vi "SetChannelVset.vi"(7 "LabVIEW Web Service Request":refnum<class "Web Request.lvclass">) -> ()   [LabVIEW 2018]
uses:
  <vilib>/wsapi/Web Request.lvclass
  subvis/Channel Properties.ctl
  CAEN globals.vi
panel:
  in  "error in (no error)":errorcluster
  # "Use the Web Service Request input terminal to call the VIs on the Web Services palette. Do not remove it from the connector pane unless you don't need access to the palette."
  # "Each additional control wired to the connector pane will be available as an input in the URL. To include an indicator in terminal-mode output (the default setting), it must also be wired to the connector pane."
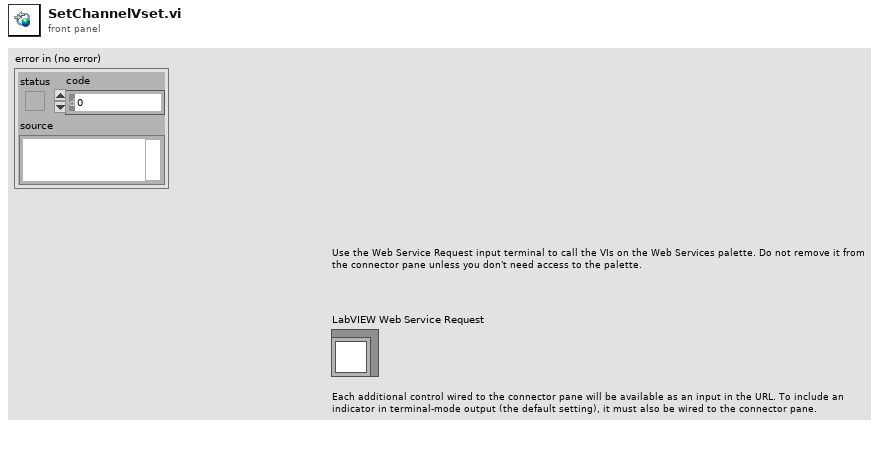
[diagram p1: front panel]
types:
  T1 = typedef "Channel Properties.ctl" = enum16{"Name", "Vset", "Vfile", "Vswmax", "Iset", "Enable", "Flag", "Vbackup"}
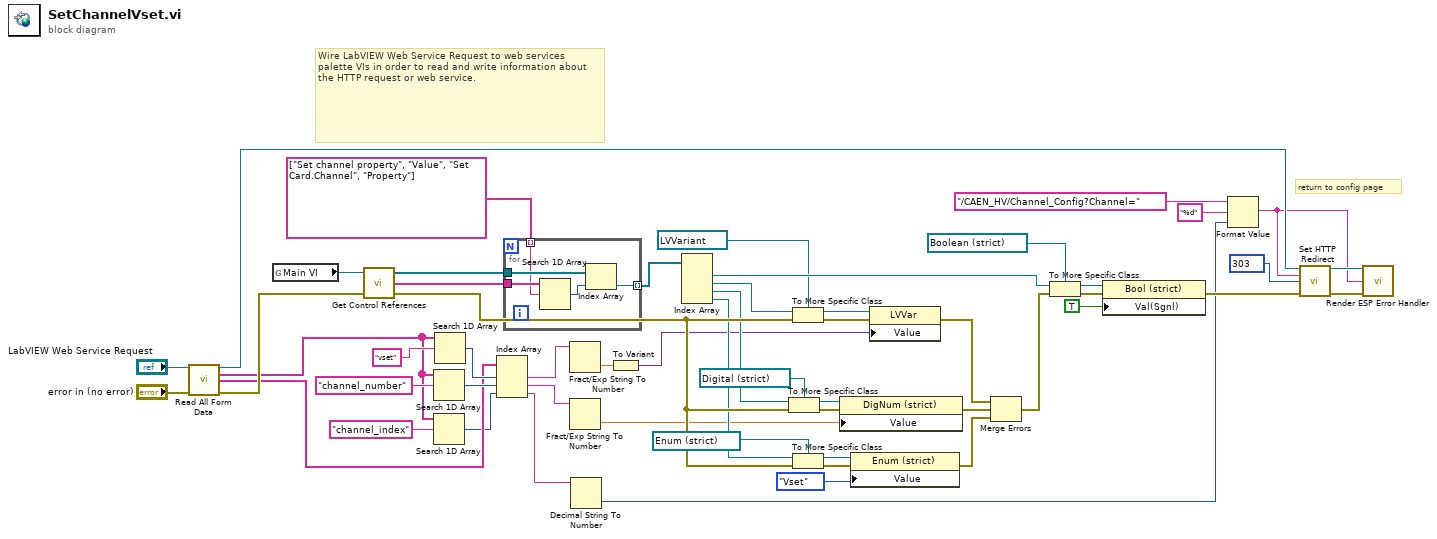
[diagram p0: block diagram]
diagram:
  w49 = 303 items=["100"=100, "101"=101, "200"=200, "201"=201, "202"=202, "203"=203, "204"=204, "205"=205, "206"=206, "300"=300, "301"=301, "302"=302, "303"=303, "304"=304, "305"=305, "306"=306, "307"=307, "400"=400, "401"=401, "402"=402, "403"=403, "404"=404, "405"=405, "406"=406, "407"=407, "408"=408, "409"=409, "410"=410, "411"=411, "412"=412, "413"=413, "414"=414, "415"=415, "416"=416, "417"=417, "500"=500, "501"=501, "502"=502, "503"=503, "504"=504, "505"=505] ("response code (307)")
  # "return to config page"
  # "Wire LabVIEW Web Service Request to web services palette VIs in order to read and write information about the HTTP request or web service."
  n1 = call <vilib>:"Read All Form Data.vi"("LabVIEW Web Service Request"="LabVIEW Web Service Request", "error in (no error)"="error in (no error)") -> ("LabVIEW Web Service Request out"=w25:refnum<class "Web Request.lvclass">, "Key"=w6:string[], "Value"=w17:string[], "error out"=w26:errorcluster)  [unwired: 9 in, 1 out]
  n2 = global read "CAEN globals.vi" "Main VI"() -> (w54:refnum<vi>)
  n3 = call "Get Control References.vi"("error in"=w26, "This vi"=w54) -> ("error out"=w28:errorcluster, "Control Names"=w53:string[], "Controls[]"=w52:refnum<vi>[])  [unwired: 1 in]
  n4 = Search 1D Array(1D array=w6, element="channel_number") -> (index of element=w44:i32)  [unwired: 1 in]
  n5 = Search 1D Array(1D array=w6, element="channel_index") -> (index of element=w5:i32)  [unwired: 1 in]
  n6 = Search 1D Array(1D array=w6, element="vset") -> (index of element=w45:i32)  [unwired: 1 in]
  n7 = Index Array(array=w17, index #1=w45, index #2=w44, index #3=w5) -> (element #1=w16:string, element #2=w13:string, element #3=w4:string)
  n8 = for {
    tunnel: w53 -> [w59]
    tunnel: w52 -> [w58]
    tunnel: [w56] -> w23 mode=indexing
    tunnel: string[] ["Set channel property", "Value", "Set Card.Channel", "Property"] ("Control Names") -> [w55] mode=indexing
    n9 = Search 1D Array(1D array=w59, element=w55) -> (index of element=w57:i32)  [unwired: 1 in]
    n10 = Index Array(array=w58, index=w57) -> (element=w56:refnum<vi>)
  }
  n11 = Fract/Exp String To Number(string=w16) -> (number=w15:dbl)  [unwired: 3 in, 1 out]
  n12 = Fract/Exp String To Number(string=w13) -> (number=w10:dbl)  [unwired: 3 in, 1 out]
  n13 = Decimal String To Number(string=w4) -> (number=w3:i32)  [unwired: 2 in, 1 out]
  n14 = To Variant(anything=w15) -> (Variant=w14:variant)
  n15 = Index Array(array=w23) -> (element #1=w22:refnum<vi>, element #2=w21:refnum<vi>, element #3=w20:refnum<vi>, element #4=w19:refnum<vi>)  [unwired: 4 in]
  n16 = To More Specific Class(target class=refnum<vi> refnum ("number"), reference=w20, error in=w28) -> (specific class reference=w41:refnum<vi>, error out=w40:errorcluster)
  n17 = To More Specific Class(target class=refnum<vi> refnum ("Value"), reference=w21, error in=w28) -> (specific class reference=w50:refnum<vi>, error out=w51:errorcluster)
  n18 = To More Specific Class(target class=refnum<vi> refnum ("Value (Signaling)"), reference=w19, error in=w28) -> (specific class reference=w38:refnum<vi>, error out=w39:errorcluster)
  n19 = property class="DigNum (strict)"(reference=w41, error in=w40, "Value"=w10) -> (error out=w31:errorcluster)  [unwired: 1 out]
  n20 = property class="Enum (strict)"(reference=w38, error in=w39, "Value"=Channel_Properties."Vset" ("Value (Signaling)")) -> (error out=w32:errorcluster)  [unwired: 1 out]
  n21 = property class="LVVar"(reference=w50, error in=w51, "Value"=w14) -> (error out=w30:errorcluster)  [unwired: 1 out]
  n22 = Merge Errors(w30, w31, w32) -> (w29:errorcluster)
  n23 = To More Specific Class(target class=refnum<vi> refnum ("replace all? (F)"), reference=w22, error in=w29) -> (specific class reference=w36:refnum<vi>, error out=w35:errorcluster)
  n24 = property class="Bool (strict)"(reference=w36, error in=w35, "Val(Sgnl)"=TRUE ("Value (Signaling)")) -> (error out=w33:errorcluster)  [unwired: 1 out]
  n25 = Format Value(string ("")="/CAEN_HV/Channel_Config?Channel=" ("redirect URL"), format string="%d", value (0)=w3) -> (output string=w11:string)
  n26 = call <vilib>:"Set HTTP Redirect.vi"("LabVIEW Web Service Request"=w25, "redirect URL"=w11, "response code (307)"=w49, "error in (no error)"=w33) -> ("LabVIEW Web Service Request out"=w47:refnum<class "Web Request.lvclass">, "error out"=w48:errorcluster)  [unwired: 10 in]
  n27 = call "Render ESP Error Handler.vi"("LabVIEW Web Service Request"=w47, "Link"=w11, "error in (no error)"=w48) -> ()  [unwired: 11 in, 2 out]
